vi "LVClass_WavefrontCorrector Check to Actuator Absolute Position.vi"(0 "WavefrontCorrector in":refnum<class "WavefrontCorrector.lvclass">, 5 "Index of actuator":i32, 7 "Position":sgl, 11 "error in (no error)":errorcluster) -> (4 "WavefrontCorrector out":refnum<class "WavefrontCorrector.lvclass">, 15 "error out":errorcluster)   [LabVIEW 2020, in "WavefrontCorrector.lvclass"]
doc: "<B>correctorIn</B> : WavefrontCorrector object.\n<B>correctorOut</B> : WavefrontCorrector object.\n<B>actuator_index</B> : Index of the actuator.\n<B>position</B> : Requested absolutes positions."
uses:
  WavefrontCorrector.lvclass
  WavefrontCorrector.lvclass/WavefrontCorrector.ctl
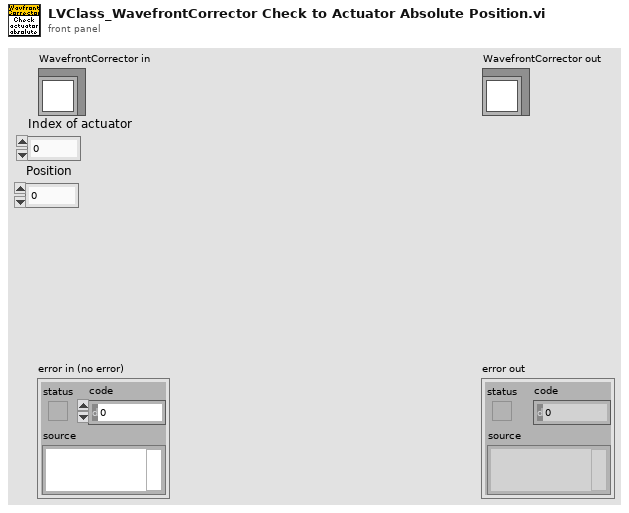
[diagram p1: front panel]
types:
  T1 = typedef "ClassID.ctl" = i64
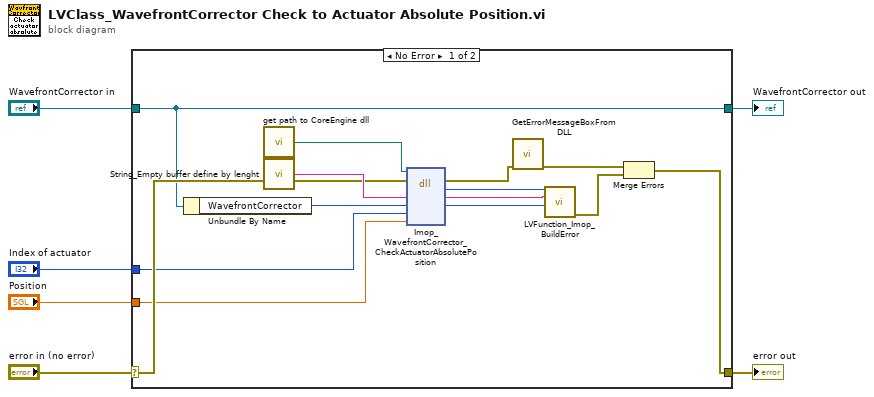
[diagram p0: block diagram]
diagram:
  n1 = case shown="No Error" "error in (no error)" {
    selector: "error in (no error)" -> [w18 w22]
    tunnel: [w10 w22] -> w5
    tunnel: [w9 w21] -> w3
    tunnel: "WavefrontCorrector in" -> [w9 w21]
    tunnel: "Index of actuator" -> [w17 _]
    tunnel: "Position" -> [w16 _]
    frame No Error {
      n2 = Unbundle By Name(w9) -> ("WavefrontCorrector"=w8:T1)
      n3 = call "get path to CoreEngine dll.vi"() -> ("path to wavekit library"=w20:path)  [unwired: 14 in, 1 out]
      n4 = call "String_Empty buffer define by lenght.vi"() -> ("Empty buffer"=w19:string)  [unwired: 1 in]
      n5 = dll-call lib="D:/FLE/0.Code/CoreEngine4_Suite/LV2011_interface/DLLs/c_interface_vc100.dll" fn="Imop_WavefrontCorrector_CheckActuatorAbsolutePosition"(path in=w20, error in=w18, "Message"=w19, "WavefrontCorrector"=w8, "Index of actuator"=w17, "Position"=w16) -> (error out=w15:errorcluster, "return type"=w12:i32, "Message"=w11:string, "WavefrontCorrector"=w7:i64)  [unwired: 3 in, 1 out]
      n6 = call "GetErrorMessageBoxFromDLL.vi"("error IN"=w15) -> ("error OUT"=w14:errorcluster)  [unwired: 10 in]
      n7 = call "LVFunction_Imop_BuildError.vi"("code"=w12, "String to Prepend to source (\"\")"=w11, "Adresse"=w7) -> ("error out"=w13:errorcluster)  [unwired: 12 in]
      n8 = Merge Errors(w14, w13) -> (w10:errorcluster)
    }
    frame Error {
    }
  }
  "error out" <- w5
  "WavefrontCorrector out" <- w3
